vi "Autonomous Independent.vi"() -> ()   [LabVIEW 2016]
doc: "This VI is called when autonomous begins, and will automatically be terminated when autonomous ends. You can carry out timed or sensor driven robot movement independently without needing to return to the caller."
uses:
  <vilib>/Rock Robotics/WPI/Utilities/WPI_GetSetVariantRefNum.vi
  <vilib>/Rock Robotics/Network Tables/NT Write Numeric Array.vi
  <vilib>/Rock Robotics/Network Tables/NT Read String.vi
  <vilib>/addons/control/pid/pid.llb/PID (DBL).vi
  <vilib>/Rock Robotics/WPI/RobotDrive/WPI_RobotDriveMecanumDrive_Cartesian.vi
  <vilib>/addons/control/pid/NI_PID_pid.lvlib
panel:
  out "Yaw":dbl=2.26
  out "Data":T1(graph)={"setpoint"=0.0, "Yaw"=2.26, "dt out (s)"=0.0010000000474974513}
  in  "setpoint":dbl(slide) scale=-50.0..50.0
  in  "PID gains":T2={"proportional gain (Kc)"=1.0, "integral time (Ti, min)"=0.01, "derivative time (Td, min)"=0.0} {"derivative time (Td, min)" scale=0.0..0.05; "integral time (Ti, min)" scale=0.0..0.00243; "proportional gain (Kc)" scale=0.0..0.284195}
  out "proportional gain (Kc)":dbl=1.0
  out "integral time (Ti, min)":dbl=0.01
  out "derivative time (Td, min)":dbl
  in  "speed":dbl(slide)=0.10126903553299492 scale=-0.15..0.15
  out "x .or. y?":bool=TRUE
  out "s? t:f":dbl=0.9
  out "Right":dbl(graph)=69.75220843172497
  out "Right":dbl=69.75220843172497
  out "Left":dbl(graph)=57.45456942754214
  out "Current Movement, for debugging":T3 {"Z Joystick Value" scale=-1.0..1.0; "Y Joystick Value" scale=1.0..-1.0; "X Joystick Value" scale=-1.0..1.0}
  in  "Array of robot movements":T4(array[cluster])=[{"X Joystick Value"=-0.010101010101010017, "Y Joystick Value"=0.0, "Z Joystick Value"=0.4574773480918073, "Delay (sec)"=0.0, "Movement Name"=""}, {"X Joystick Value"=0.050505050505050594, "Y Joystick Value"=0.0, "Z Joystick Value"=-0.25616029503917137, "Delay (sec)"=0.0, "Movement Name"=""}] {"Z Joystick Value" scale=-1.0..1.0; "Y Joystick Value" scale=1.0..-1.0; "X Joystick Value" scale=-1.0..1.0}
  # "speed"
  # "Be sure to right-click and choose Data Operations>>Make Current Value default if you want to save the array values with the VI"
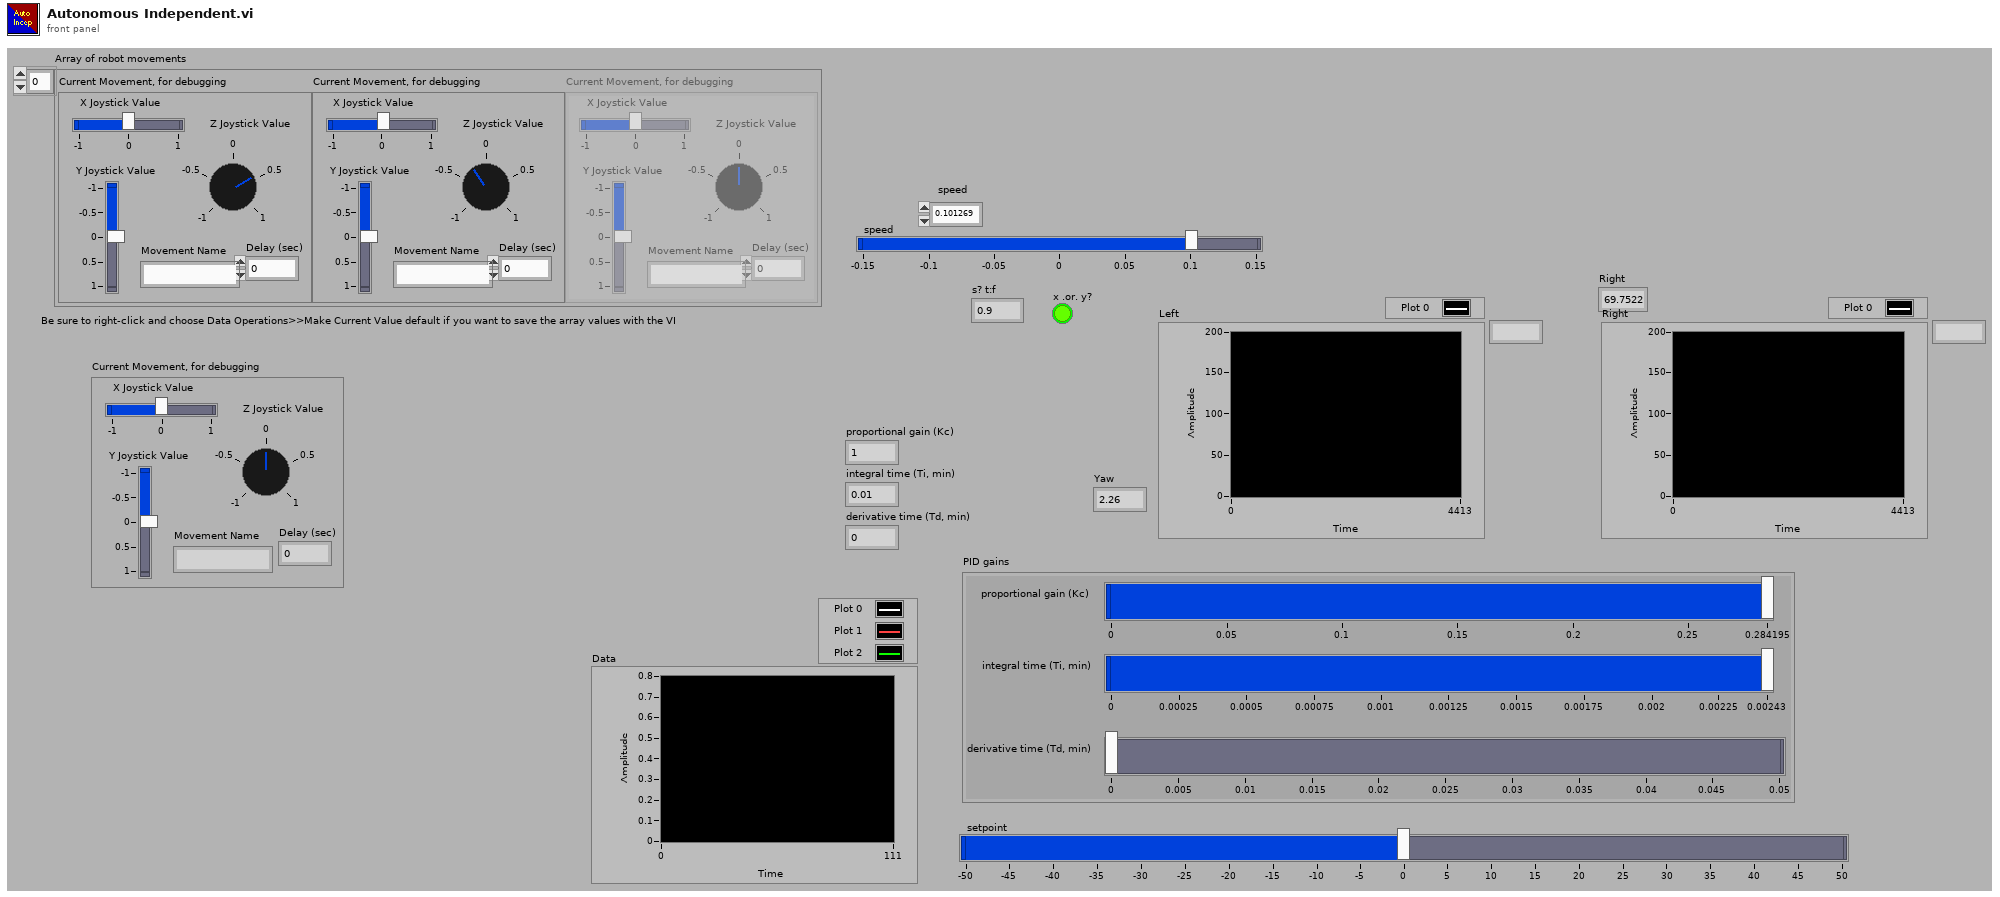
[diagram p1: front panel]
types:
  T1 = cluster{"setpoint":dbl, "Yaw":dbl, "dt out (s)":dbl}
  T2 = cluster{"proportional gain (Kc)":dbl, "integral time (Ti, min)":dbl, "derivative time (Td, min)":dbl}
  T3 = cluster{"X Joystick Value":dbl, "Y Joystick Value":dbl, "Z Joystick Value":dbl, "Delay (sec)":dbl, "Movement Name":string}
  T4 = cluster{"X Joystick Value":dbl, "Y Joystick Value":dbl, "Z Joystick Value":dbl, "Delay (sec)":dbl, "Movement Name":string}[]
  T5 = typedef "WPI_JoystickDevRef.ctl" = cluster{"Device":T6}
  T6 = typedef "WPI_JoystickDeviceEnum.ctl" = enum16{"USB 0", "USB 1", "USB 2", "USB 3", "USB 4", "USB 5"}
  T7 = typedef "WPI_AnalogChannelDevRef.ctl" = cluster{"DevStatus":errorcluster, "Analog Channel":T8}
  T8 = typedef "FPGA_AIChannel.ctl" = enum8{"AI 0", "AI 1", "AI 2", "AI 3", "AI MXP 0", "AI MXP 1", "AI MXP 2", "AI MXP 3", "Invalid"}
  T9 = typedef "WPI_RobotDriveDevRef.ctl" = cluster{"DevStatus":errorcluster, "Motors[]":T10[], "Square Inputs":bool, "Max Output":dbl}
  T10 = typedef "WPI_MotorControlDeviceRef.ctl" = cluster{"DeviceStatus":errorcluster, "Type":T11, "PWM":cluster{"PWM Channel":T12, "DeadBand":T13}, "CAN":cluster{"Device Number":u8, "SetOutput VI Ref":variant, "GetOutput VI Ref":variant, "Enable VI Ref":variant, "Disable VI Ref":variant, "Data":variant}, "Invert":bool}
  T11 = typedef "WPI_MotorControlType.ctl" = enum16{"PWM", "CAN"}
  T12 = typedef "FPGA_DIOPWMChannel.ctl" = enum8{"PWM 0", "PWM 1", "PWM 2", "PWM 3", "PWM 4", "PWM 5", "PWM 6", "PWM 7", "PWM 8", "PWM 9", "PWM MXP 0", "PWM MXP 1", "PWM MXP 2", "PWM MXP 3", "PWM MXP 4", "PWM MXP 5", "PWM MXP 6", "PWM MXP 7", "PWM MXP 8", "PWM MXP 9", "Invalid"}
  T13 = typedef "WPI_PWMDeadband.ctl" = cluster{"Name":string, "maxPositivePwm":i32, "minPositivePwm":i32, "centerPwm":i32, "maxNegativePwm":i32, "minNegativePwm":i32, "angularRange":u16}
  T14 = cluster{"Yaw":dbl, "Roll":dbl, "Pitch":dbl, "Heading":dbl, "Fused Heading":dbl}
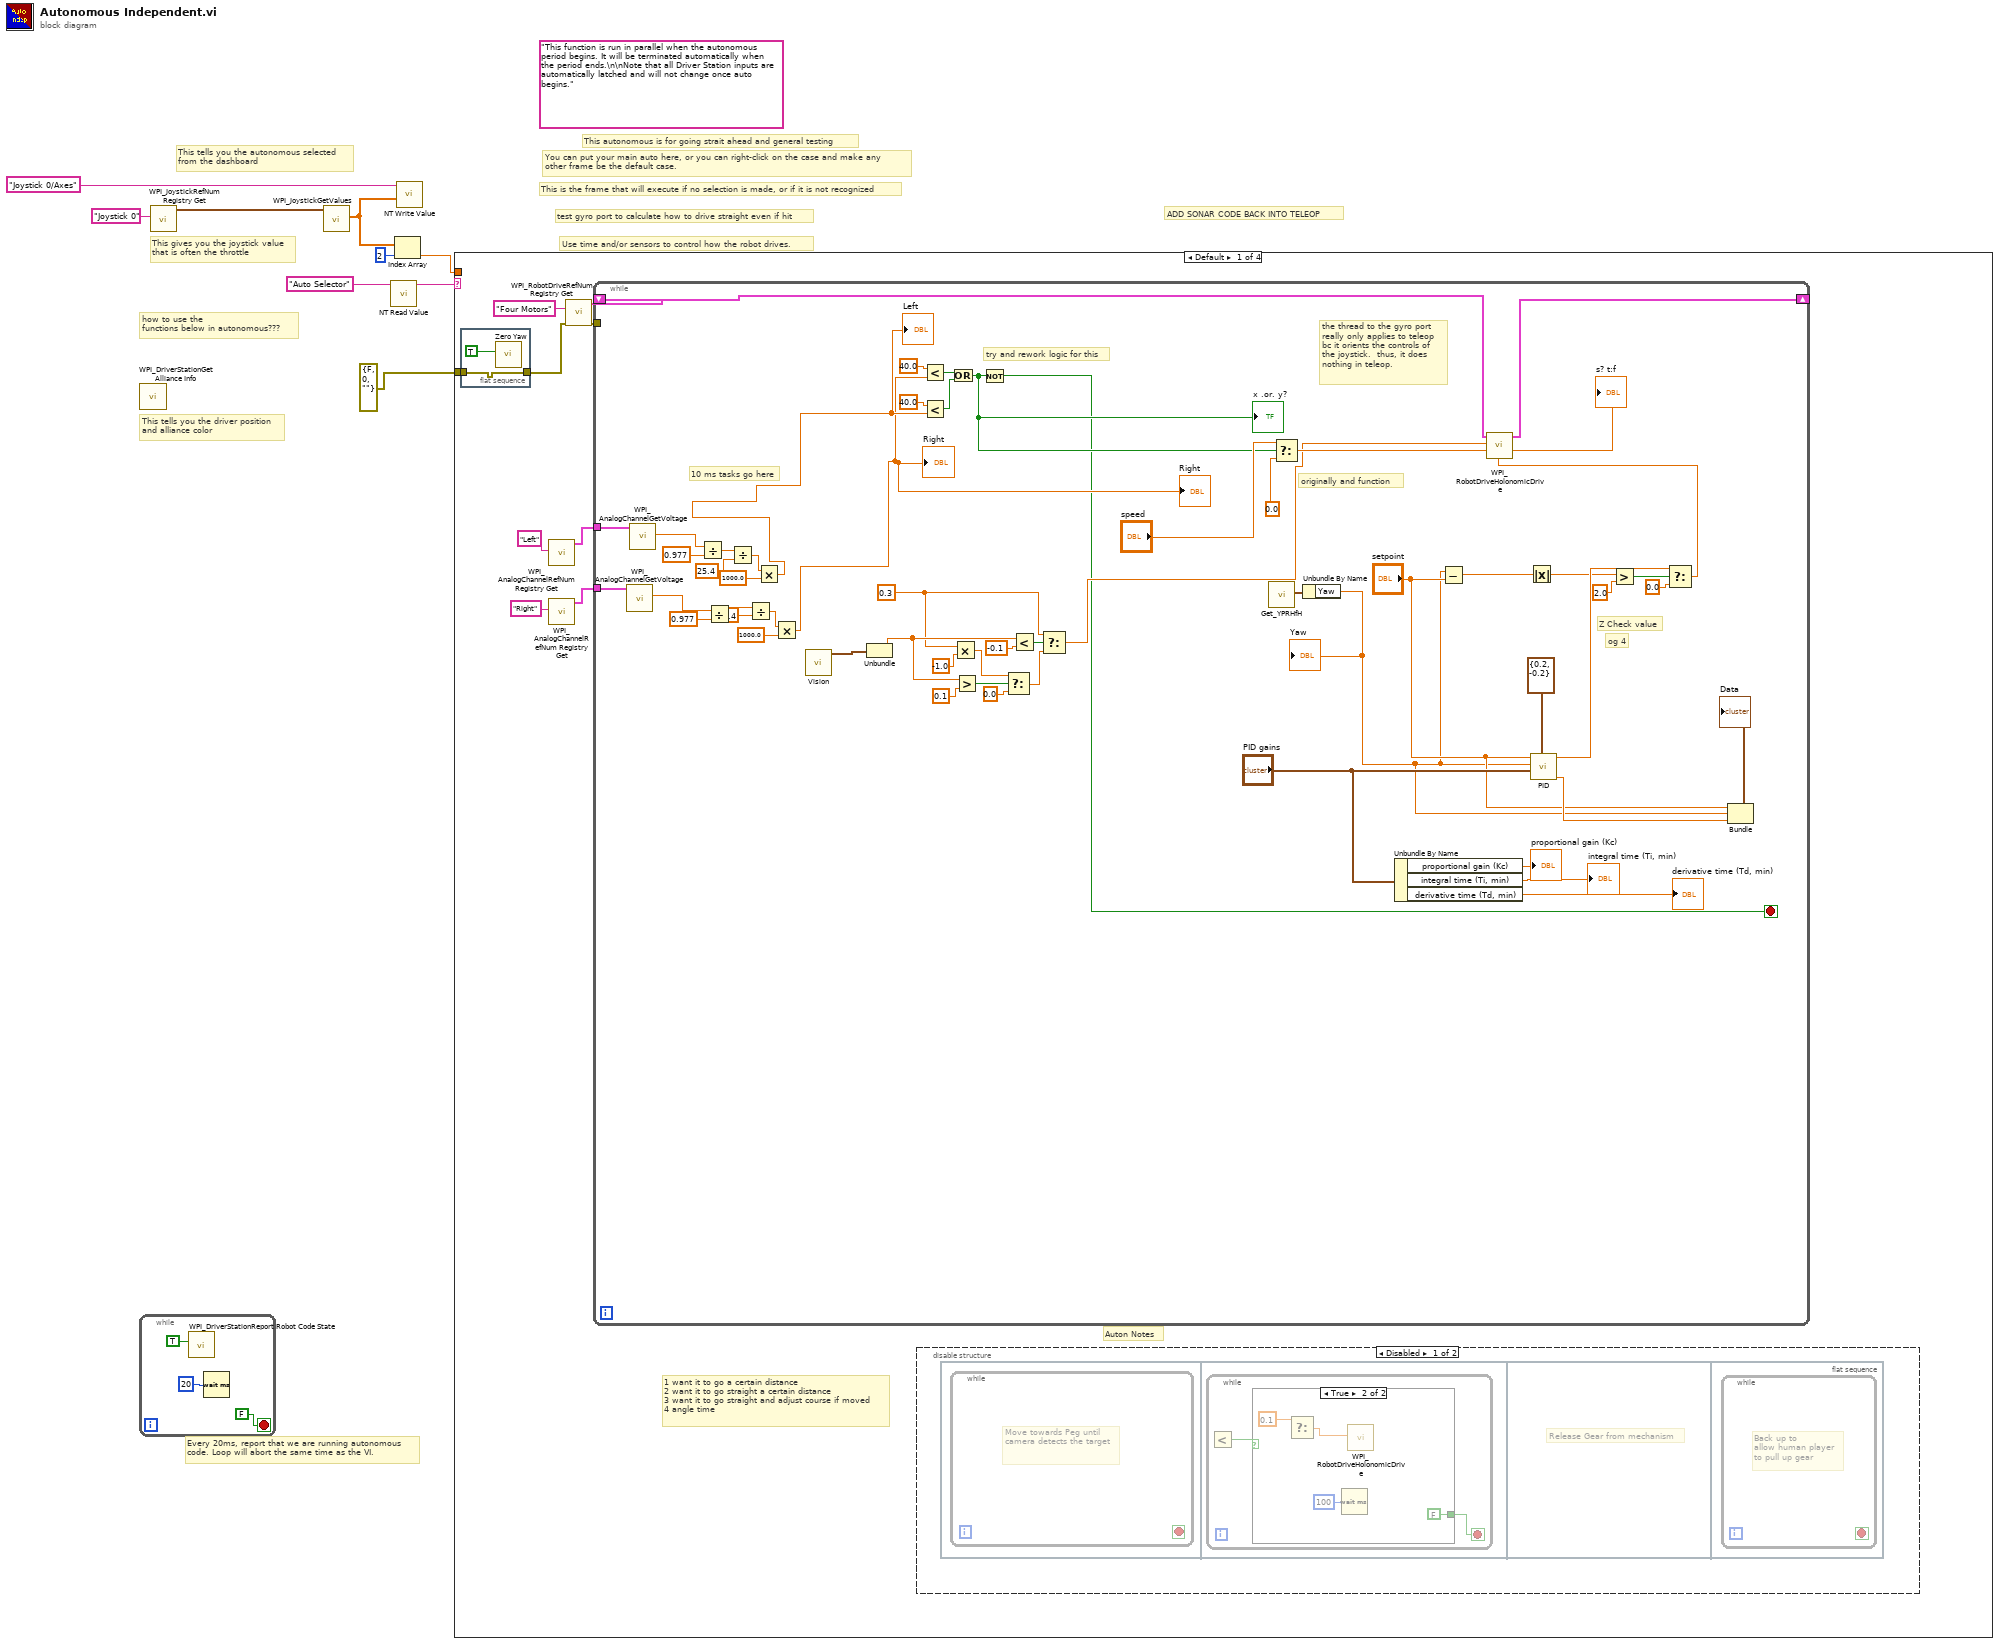
[diagram p0: block diagram]
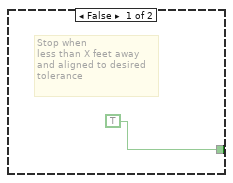
[diagram p2: hidden frame]
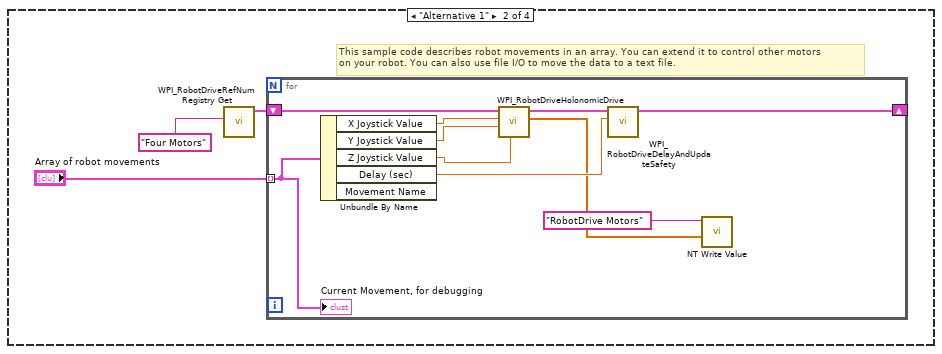
[diagram p4: hidden frame]
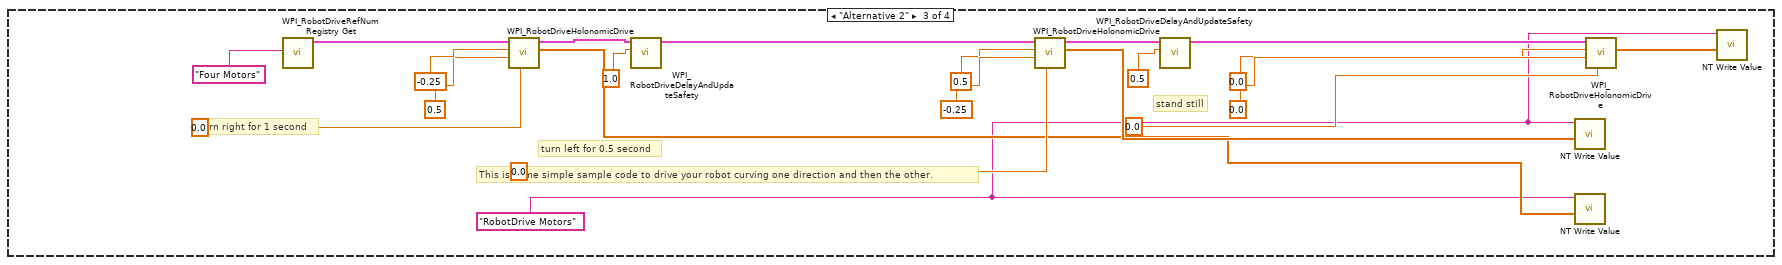
[diagram p5: hidden frame]
diagram:
  (unwired) "This function is run in parallel when the autonomous period begins. It will be terminated automatically when the period ends.\n\nNote that all Driver Station inputs are automatically latched and will not change once auto begins."
  # "ADD SONAR CODE BACK INTO TELEOP"
  # "test gyro port to calculate how to drive straight even if hit"
  # "This autonomous is for going strait ahead and general testing"
  # "You can put your main auto here, or you can right-click on the case and make any\nother frame be the default case."
  # "This is the frame that will execute if no selection is made, or if it is not recognized"
  # "how to use the\nfunctions below in autonomous???"
  # "This tells you the autonomous selected\nfrom the dashboard"
  # "Every 20ms, report that we are running autonomous\ncode. Loop will abort the same time as the VI."
  # "This gives you the joystick value\nthat is often the throttle"
  # "Use time and/or sensors to control how the robot drives."
  # "This tells you the driver position\nand alliance color"
  n1 = call <vilib>:"WPI_DriverStationGet Alliance Info.vi"() -> ()  [unwired: 12 out]
  n2 = while {
    stop <- FALSE stop-if-true
    n3 = call <vilib>:"WPI_DriverStationReport Robot Code State.vi"("Autonomous"=TRUE) -> ()  [unwired: 10 in, 1 out]
    n4 = Wait (ms)(milliseconds to wait=u32 20) -> ()  [unwired: 1 out]
  }
  n5 = call <vilib>:"WPI_JoystickRefNum Registry Get.vi"("refnum name"="Joystick 0") -> ("JoystickDevRef"=w8:T5)  [unwired: 1 in, 9 out]
  n6 = call <vilib>:"WPI_JoystickGetValues.vi"("JoystickDevRef"=w8) -> ("Axes"=w2:dbl[])  [unwired: 6 in, 4 out]
  n7 = call-poly <vilib>:"NT Read Value.vi"("Name"="Auto Selector") -> ("String"=w5:string)  [unwired: 9 in, 1 out]
  n8 = Index Array(array=w2, index=u32 2 ("milliseconds to wait")) -> (element=w4:dbl)
  n9 = call-poly <vilib>:"NT Write Value.vi"("Numeric Array"=w2, "Name"="Joystick 0/Axes") -> ()  [unwired: 9 in, 1 out]
  n10 = case shown="Default" w5 {
    tunnel: w4 -> [_ _ _ _]
    tunnel: errorcluster {"status"=FALSE, "code"=0, "source"=""} ("error in (no error)") -> [w13 _ _ _]
    frame Default {
      # "Auton Notes"
      # "1 want it to go a certain distance\n2 want it to go straight a certain distance\n3 want it to go straight and adjust course if moved\n4 angle time"
      n11 = flat-sequence {
        tunnel: [w23] -> w14
        tunnel: w13 -> [w23]
        frame #0 {
          n12 = call <vilib>:"Zero Yaw.vi"("Zero"=TRUE) -> ()  [unwired: 11 in]
        }
      }
      n13 = call <vilib>:"WPI_AnalogChannelRefNum Registry Get.vi"("refnum name"="Left") -> ("AIDeviceRef"=w17:T7)  [unwired: 9 in, 1 out]
      n14 = call <vilib>:"WPI_AnalogChannelRefNum Registry Get.vi"("refnum name"="Right") -> ("AIDeviceRef"=w16:T7)  [unwired: 9 in, 1 out]
      n15 = call <vilib>:"WPI_RobotDriveRefNum Registry Get.vi"("error in (no error)"=w14, "refnum name"="Four Motors") -> ("error out"=w15:errorcluster, "RobotDriveDevRef"=w20:T9)  [unwired: 8 out]
      n16 = while {
        shift-right: [w28] -> _
        shift-left: w20 -> [w77]
        tunnel: w17 -> [w79]
        tunnel: w16 -> [w78]
        tunnel: w15 -> [_]
        stop <- w24 stop-if-true
        w68 = 0.3 ("t")
        # "og 4"
        # "try and rework logic for this"
        # "the thread to the gyro port\nreally only applies to teleop \nbc it orients the controls of \nthe joystick.  thus, it does \nnothing in teleop."
        # "Z Check value"
        # "10 ms tasks go here"
        # "originally and function"
        n17 = call <vilib>:"WPI_AnalogChannelGetVoltage.vi"("AIDeviceRef"=w78) -> ("Voltage"=w54:dbl)  [unwired: 8 in, 2 out]
        n18 = call <vilib>:"WPI_AnalogChannelGetVoltage.vi"("AIDeviceRef"=w79) -> ("Voltage"=w48:dbl)  [unwired: 8 in, 2 out]
        n19 = Divide(x=w48, y=0.977) -> (x/y=w50:dbl)
        n20 = Divide(x=w54, y=0.977) -> (x/y=w58:dbl)
        n21 = Divide(x=w50, y=25.4) -> (x/y=w52:dbl)
        n22 = Divide(x=w58, y=25.4) -> (x/y=w56:dbl)
        n23 = Multiply(x=w52, y=1000.0) -> (x*y=w47:dbl)
        "Left" <- w47
        n24 = Multiply(x=w56, y=1000.0) -> (x*y=w46:dbl)
        "Right" <- w46
        "Right" <- w46
        n25 = call "Vision.vi"() -> ("Center"=w76:cluster{dbl, dbl})  [unwired: 11 in]
        n26 = Unbundle(w76) -> (w75:dbl)  [unwired: 1 out]
        n27 = Less?(x=40.0, y=w46) -> (x < y?=w61:bool)
        n28 = Less?(x=40.0, y=w47) -> (x < y?=w62:bool)
        n29 = Or(x=w61, y=w62) -> (x .or. y?=w60:bool)
        "x .or. y?" <- w60
        n30 = Multiply(x=w68, y=-1.0) -> (x*y=w69:dbl)
        n31 = Greater?(x=w75, y=0.1) -> (0:w26:bool)
        n32 = Not(x=w60) -> (.not. x?=w24:bool)
        n33 = Select(t=w69, s=w26, f=0.0) -> (s? t:f=w73:dbl)
        n34 = Less?(x=w75, y=-0.1) -> (x < y?=w25:bool)
        n35 = Select(t=w68, s=w25, f=w73) -> (s? t:f=w27:dbl)
        n36 = call <vilib>:"Get_YPRHfH.vi"() -> ("YRPHfH"=w38:T14)  [unwired: 11 in]
        n37 = Select(t="speed", s=w60, f=0.0) -> (s? t:f=w65:dbl)
        "s? t:f" <- w65
        n38 = Unbundle By Name(w38) -> ("Yaw"=w29:dbl)
        "Yaw" <- w29
        n39 = Unbundle By Name("PID gains") -> ("proportional gain (Kc)"=→"proportional gain (Kc)":dbl, "integral time (Ti, min)"=→"integral time (Ti, min)":dbl, "derivative time (Td, min)"=→"derivative time (Td, min)":dbl)
        n40 = Subtract(x=w29, y="setpoint") -> (x-y=w33:dbl)
        n41 = Absolute Value(x=w33) -> (abs(x)=w31:dbl)
        n42 = call-poly <vilib>:"PID.vi"("output range"=cluster{"output high":dbl, "output low":dbl} {"output high"=0.2, "output low"=-0.2}, "PID gains"="PID gains", "process variable"=w29, "setpoint"="setpoint") -> ("dt out (s)"=w39:dbl, "output"=w40:dbl)  [unwired: 6 in]
        n43 = Greater?(x=w31, y=2.0) -> (0:w34:bool)
        n44 = Select(t=w40, s=w34, f=0.0) -> (s? t:f=w30:dbl)
        n45 = call-poly <vilib>:"WPI_RobotDriveHolonomicDrive.vi"("Rotation"=w30, "Y"=w65, "X"=w27, "RobotDriveDevRef"=w77) -> ("RobotDriveDevRef"=w28:T9)  [unwired: 5 in, 2 out]
        n46 = Bundle("setpoint"="setpoint", "Yaw"=w29, "dt out (s)"=w39) -> (→"Data":T1)  [unwired: 1 in]
      }
      n47 = disable-structure shown="Disabled" {
        frame Disabled {
          n48 = flat-sequence {
            frame #0 {
              n49 = while {
                stop <- _ stop-if-true
                # "Move towards Peg until\ncamera detects the target"
              }
            }
            frame #1 {
              n50 = while {
                stop <- w80 stop-if-true
                n51 = Less?() -> (x < y?=w81:bool)  [unwired: 2 in]
                n52 = case shown="True" w81 {
                  tunnel: [TRUE FALSE] -> w80
                  frame False {
                    # "Stop when \nless than X feet away\nand aligned to desired \ntolerance"
                  }
                  frame True {
                    n53 = Select(t=0.1) -> (s? t:f=w84:dbl)  [unwired: 2 in]
                    n54 = Wait (ms)(milliseconds to wait=u32 100) -> ()  [unwired: 1 out]
                    n55 = call-poly <vilib>:"WPI_RobotDriveHolonomicDrive.vi"("X"=w84) -> ()  [unwired: 8 in, 3 out]
                  }
                }
              }
            }
            frame #2 {
              # "Release Gear from mechanism"
            }
            frame #3 {
              n56 = while {
                stop <- _ stop-if-true
                # "Back up to \nallow human player\nto pull up gear"
              }
            }
          }
        }
        frame Enabled {
        }
      }
    }
    frame "Alternative 1" {
      # "This sample code describes robot movements in an array. You can extend it to control other motors\non your robot. You can also use file I/O to move the data to a text file."
      n57 = call <vilib>:"WPI_RobotDriveRefNum Registry Get.vi"("refnum name"="Four Motors") -> ("RobotDriveDevRef"=w88:T9)  [unwired: 1 in, 9 out]
      n58 = for {
        shift-right: [w97] -> _
        shift-left: w88 -> [w98]
        tunnel: "Array of robot movements" -> [w93] mode=indexing
        n59 = Unbundle By Name(w93) -> ("X Joystick Value"=w96:dbl, "Y Joystick Value"=w95:dbl, "Z Joystick Value"=w92:dbl, "Delay (sec)"=w94:dbl)  [unwired: 1 out]
        n60 = call-poly <vilib>:"WPI_RobotDriveHolonomicDrive.vi"("Rotation"=w92, "Y"=w95, "X"=w96, "RobotDriveDevRef"=w98) -> ("Motor Values"=w90:dbl[], "RobotDriveDevRef"=w99:T9)  [unwired: 5 in, 1 out]
        n61 = call <vilib>:"WPI_RobotDriveDelayAndUpdateSafety.vi"("Delay (s)"=w94, "RobotDriveDevRef"=w99) -> ("RobotDriveDevRef 2"=w97:T9)  [unwired: 8 in, 1 out]
        n62 = call-poly <vilib>:"NT Write Value.vi"("Numeric Array"=w90, "Name"="RobotDrive Motors") -> ()  [unwired: 9 in, 1 out]
        "Current Movement, for debugging" <- w93
      }
    }
    frame "Alternative 2" {
      w100 = "RobotDrive Motors" ("Name")
      # "This is some simple sample code to drive your robot curving one direction and then the other."
      # "stand still"
      # "turn left for 0.5 second"
      # "turn right for 1 second"
      n63 = call <vilib>:"WPI_RobotDriveRefNum Registry Get.vi"("refnum name"="Four Motors") -> ("RobotDriveDevRef"=w117:T9)  [unwired: 1 in, 9 out]
      n64 = call-poly <vilib>:"WPI_RobotDriveHolonomicDrive.vi"("Rotation"=0.0, "Y"=0.5 ("X axis value"), "X"=-0.25 ("X axis value"), "RobotDriveDevRef"=w117) -> ("Motor Values"=w101:dbl[], "RobotDriveDevRef"=w110:T9)  [unwired: 5 in, 1 out]
      n65 = call <vilib>:"WPI_RobotDriveDelayAndUpdateSafety.vi"("Delay (s)"=1.0, "RobotDriveDevRef"=w110) -> ("RobotDriveDevRef 2"=w111:T9)  [unwired: 8 in, 1 out]
      n66 = call-poly <vilib>:"WPI_RobotDriveHolonomicDrive.vi"("Rotation"=0.0, "Y"=-0.25 ("X axis value"), "X"=0.5 ("X axis value"), "RobotDriveDevRef"=w111) -> ("Motor Values"=w102:dbl[], "RobotDriveDevRef"=w112:T9)  [unwired: 5 in, 1 out]
      n67 = call <vilib>:"WPI_RobotDriveDelayAndUpdateSafety.vi"("Delay (s)"=0.5, "RobotDriveDevRef"=w112) -> ("RobotDriveDevRef 2"=w113:T9)  [unwired: 8 in, 1 out]
      n68 = call-poly <vilib>:"NT Write Value.vi"("Numeric Array"=w102, "Name"=w100) -> ()  [unwired: 9 in, 1 out]
      n69 = call-poly <vilib>:"NT Write Value.vi"("Numeric Array"=w101, "Name"=w100) -> ()  [unwired: 9 in, 1 out]
      n70 = call-poly <vilib>:"WPI_RobotDriveHolonomicDrive.vi"("Rotation"=0.0 ("X axis value"), "Y"=0.0 ("X axis value"), "X"=0.0 ("X axis value"), "RobotDriveDevRef"=w113) -> ("Motor Values"=w103:dbl[])  [unwired: 5 in, 2 out]
      n71 = call-poly <vilib>:"NT Write Value.vi"("Numeric Array"=w103, "Name"=w100) -> ()  [unwired: 9 in, 1 out]
    }
    frame "Your Turn" {
    }
  }
